vi "TCP SSH.vi"(6 "States":T1, 7 "Error In":errorcluster) -> (0 "Error  Out":errorcluster, 2 "Response":string)   [LabVIEW 2021]
uses:
  TCP states.ctl
  <vilib>/Field R&D Services/LIBSSH2 for LabVIEW/Toolkit/Session/Support/Create from SSH.vi
  <vilib>/Field R&D Services/LIBSSH2 for LabVIEW/Toolkit/Session/Support/Password Authentication.vi
  <vilib>/Field R&D Services/LIBSSH2 for LabVIEW/Toolkit/Channel/Support/Create from Session.vi
  <vilib>/Field R&D Services/LIBSSH2 for LabVIEW/Toolkit/Channel/Support/Destroy to Session.vi
  <vilib>/Field R&D Services/LIBSSH2 for LabVIEW/Toolkit/Session/Support/Destroy to SSH.vi
  <vilib>/Field R&D Services/LIBSSH2 for LabVIEW/Toolkit/Channel/Channel.lvclass
  <vilib>/Field R&D Services/LIBSSH2 for LabVIEW/Toolkit/SSH/SSH.lvclass
  <vilib>/Field R&D Services/LIBSSH2 for LabVIEW/Toolkit/Session/Session.lvclass
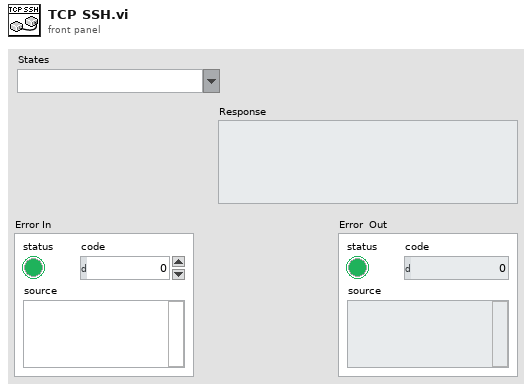
[diagram p1: front panel]
types:
  T1 = typedef "TCP states.ctl" = string
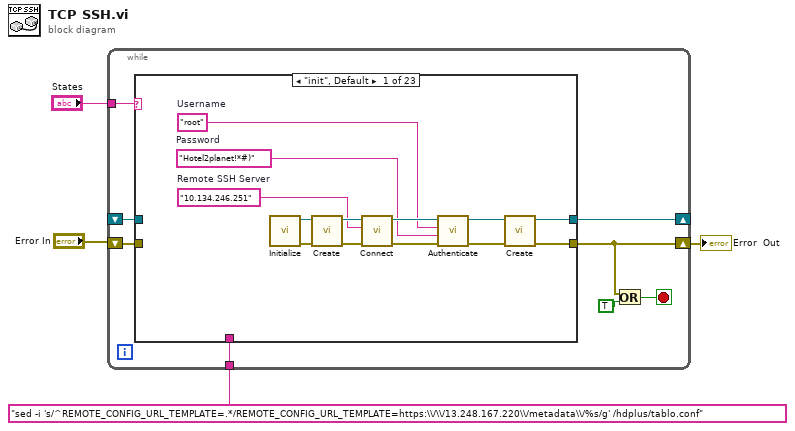
[diagram p0: block diagram]
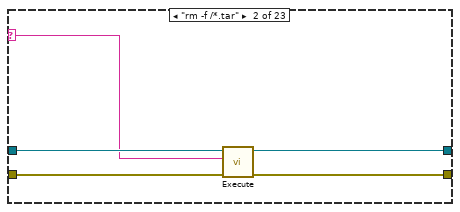
[diagram p2: hidden frame]
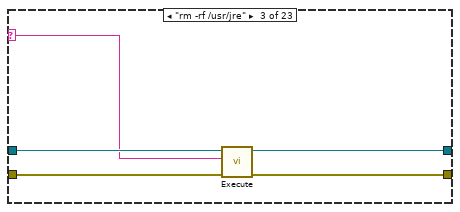
[diagram p3: hidden frame]
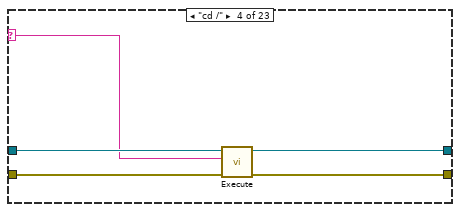
[diagram p4: hidden frame]
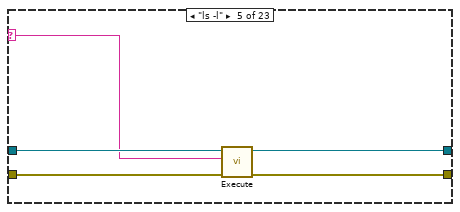
[diagram p5: hidden frame]
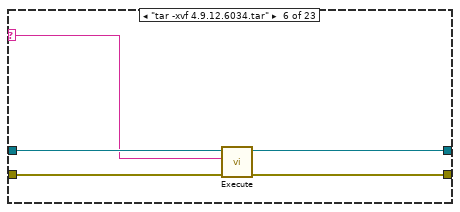
[diagram p6: hidden frame]
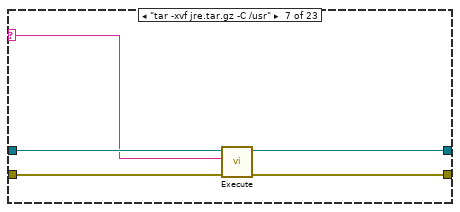
[diagram p7: hidden frame]
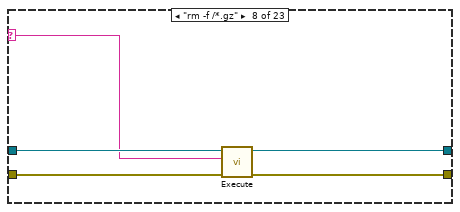
[diagram p8: hidden frame]
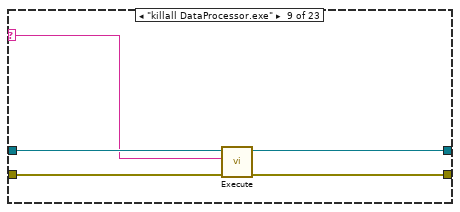
[diagram p9: hidden frame]
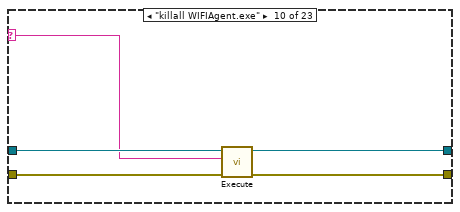
[diagram p10: hidden frame]
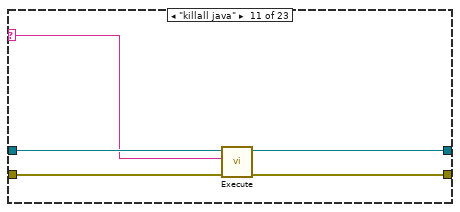
[diagram p11: hidden frame]
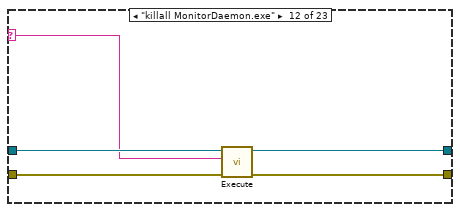
[diagram p12: hidden frame]
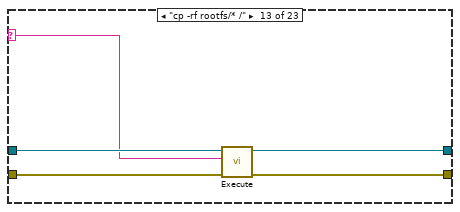
[diagram p13: hidden frame]
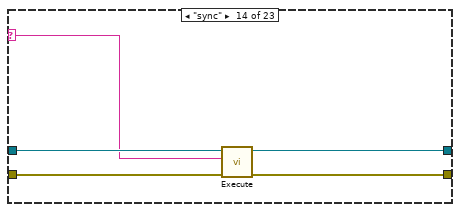
[diagram p14: hidden frame]
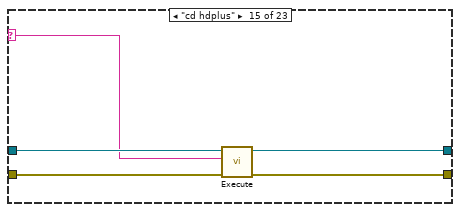
[diagram p15: hidden frame]
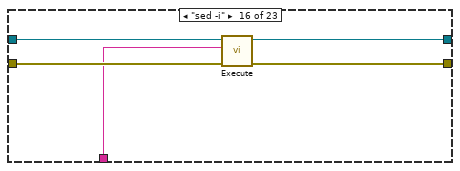
[diagram p16: hidden frame]
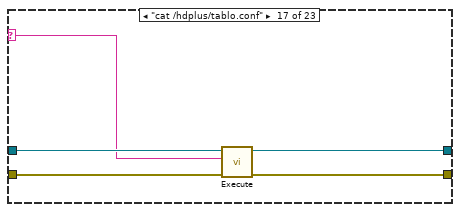
[diagram p17: hidden frame]
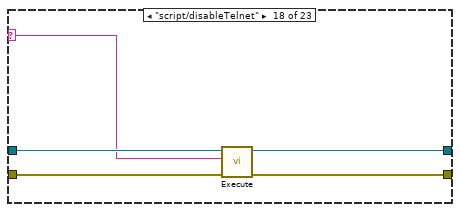
[diagram p18: hidden frame]
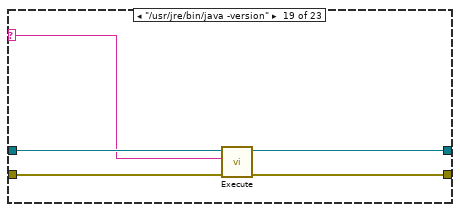
[diagram p19: hidden frame]
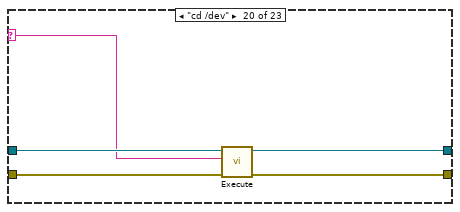
[diagram p20: hidden frame]
diagram:
  n1 = while {
    tunnel: "States" -> [w12]
    shift-right: [w10] -> _
    shift-left: _ -> [w11]
    shift-right: [w8] -> w2
    shift-left: "Error In" -> [w9]
    tunnel: "sed -i 's/^REMOTE_CONFIG_URL_TEMPLATE=.*/REMOTE_CONFIG_URL_TEMPLATE=https:\\/\\/13.248.167.220\\/metadata\\/%s/g' /hdplus/tablo.conf" ("Command") -> [w5]
    stop <- w6 stop-if-true
    n2 = case shown="\"init\", Default" w12 {
      selector: w12 -> [_ w28 w33 w38 w43 w48 w53 w58 w63 w68 w73 w78 w83 w88 w93 _ w101 w106 w111 w116 w121 _ _]
      tunnel: w11 -> [_ w30 w35 w40 w45 w50 w55 w60 w65 w70 w75 w80 w85 w90 w95 w100 w105 w110 w115 w120 w125 w128 w135]
      tunnel: [w15 w29 w32 w37 w42 w47 w52 w57 w62 w67 w72 w77 w82 w87 w92 w98 w103 w108 w113 w118 w123 w126 _] -> w10
      tunnel: [w13 w26 w31 w36 w41 w46 w51 w56 w61 w66 w71 w76 w81 w86 w91 w97 w102 w107 w112 w117 w122 w127 w133] -> w8
      tunnel: w9 -> [_ w27 w34 w39 w44 w49 w54 w59 w64 w69 w74 w79 w84 w89 w94 w99 w104 w109 w114 w119 w124 w129 w134]
      tunnel: w5 -> [_ _ _ _ _ _ _ _ _ _ _ _ _ _ _ w96 _ _ _ _ _ _ _]
      frame "init", Default {
        w17 = "10.134.246.251"  # Remote SSH Server
        w19 = "Hotel2planet!*#)"  # Password
        w18 = "root"  # Username
        n3 = call <vilib>:"Initialize.vi"() -> ("Error Out"=w21:errorcluster, "SSH"=w20:refnum<class "SSH.lvclass">)  [unwired: 10 in]
        n4 = call-poly <vilib>:"Create.vi"("Error In"=w21, "SSH"=w20) -> ("Error Out"=w23:errorcluster, "Sesssion"=w22:refnum<class "Session.lvclass">)  [unwired: 8 in]
        n5 = call <vilib>:"Connect.vi"("Error In"=w23, "Address"=w17, "Session In"=w22) -> ("Error Out"=w25:errorcluster, "Sesssion Out"=w24:refnum<class "Session.lvclass">)  [unwired: 7 in]
        n6 = call-poly <vilib>:"Authenticate.vi"("Error In"=w25, "Password"=w19, "Username"=w18, "Session In"=w24) -> ("Error Out"=w14:errorcluster, "Sesssion Out"=w16:refnum<class "Session.lvclass">)  [unwired: 6 in]
        n7 = call-poly <vilib>:"Create.vi"("Error In"=w14, "Session"=w16) -> ("Error Out"=w13:errorcluster, "Channel"=w15:refnum<class "Channel.lvclass">)  [unwired: 8 in]
      }
      frame "rm -f /*.tar" {
        n8 = call <vilib>:"Execute.vi"("Error In"=w27, "Command"=w28, "Channel In"=w30) -> ("Error Out"=w26:errorcluster, "Channel Out"=w29:refnum<class "Channel.lvclass">)  [unwired: 7 in]
      }
      frame "rm -rf /usr/jre" {
        n9 = call <vilib>:"Execute.vi"("Error In"=w34, "Command"=w33, "Channel In"=w35) -> ("Error Out"=w31:errorcluster, "Channel Out"=w32:refnum<class "Channel.lvclass">)  [unwired: 7 in]
      }
      frame "cd /" {
        n10 = call <vilib>:"Execute.vi"("Error In"=w39, "Command"=w38, "Channel In"=w40) -> ("Error Out"=w36:errorcluster, "Channel Out"=w37:refnum<class "Channel.lvclass">)  [unwired: 7 in]
      }
      frame "ls -l" {
        n11 = call <vilib>:"Execute.vi"("Error In"=w44, "Command"=w43, "Channel In"=w45) -> ("Error Out"=w41:errorcluster, "Channel Out"=w42:refnum<class "Channel.lvclass">)  [unwired: 7 in]
      }
      frame "tar -xvf 4.9.12.6034.tar" {
        n12 = call <vilib>:"Execute.vi"("Error In"=w49, "Command"=w48, "Channel In"=w50) -> ("Error Out"=w46:errorcluster, "Channel Out"=w47:refnum<class "Channel.lvclass">)  [unwired: 7 in]
      }
      frame "tar -xvf jre.tar.gz -C /usr" {
        n13 = call <vilib>:"Execute.vi"("Error In"=w54, "Command"=w53, "Channel In"=w55) -> ("Error Out"=w51:errorcluster, "Channel Out"=w52:refnum<class "Channel.lvclass">)  [unwired: 7 in]
      }
      frame "rm -f /*.gz" {
        n14 = call <vilib>:"Execute.vi"("Error In"=w59, "Command"=w58, "Channel In"=w60) -> ("Error Out"=w56:errorcluster, "Channel Out"=w57:refnum<class "Channel.lvclass">)  [unwired: 7 in]
      }
      frame "killall DataProcessor.exe" {
        n15 = call <vilib>:"Execute.vi"("Error In"=w64, "Command"=w63, "Channel In"=w65) -> ("Error Out"=w61:errorcluster, "Channel Out"=w62:refnum<class "Channel.lvclass">)  [unwired: 7 in]
      }
      frame "killall WIFIAgent.exe" {
        n16 = call <vilib>:"Execute.vi"("Error In"=w69, "Command"=w68, "Channel In"=w70) -> ("Error Out"=w66:errorcluster, "Channel Out"=w67:refnum<class "Channel.lvclass">)  [unwired: 7 in]
      }
      frame "killall java" {
        n17 = call <vilib>:"Execute.vi"("Error In"=w74, "Command"=w73, "Channel In"=w75) -> ("Error Out"=w71:errorcluster, "Channel Out"=w72:refnum<class "Channel.lvclass">)  [unwired: 7 in]
      }
      frame "killall MonitorDaemon.exe" {
        n18 = call <vilib>:"Execute.vi"("Error In"=w79, "Command"=w78, "Channel In"=w80) -> ("Error Out"=w76:errorcluster, "Channel Out"=w77:refnum<class "Channel.lvclass">)  [unwired: 7 in]
      }
      frame "cp -rf rootfs/* /" {
        n19 = call <vilib>:"Execute.vi"("Error In"=w84, "Command"=w83, "Channel In"=w85) -> ("Error Out"=w81:errorcluster, "Channel Out"=w82:refnum<class "Channel.lvclass">)  [unwired: 7 in]
      }
      frame "sync" {
        n20 = call <vilib>:"Execute.vi"("Error In"=w89, "Command"=w88, "Channel In"=w90) -> ("Error Out"=w86:errorcluster, "Channel Out"=w87:refnum<class "Channel.lvclass">)  [unwired: 7 in]
      }
      frame "cd hdplus" {
        n21 = call <vilib>:"Execute.vi"("Error In"=w94, "Command"=w93, "Channel In"=w95) -> ("Error Out"=w91:errorcluster, "Channel Out"=w92:refnum<class "Channel.lvclass">)  [unwired: 7 in]
      }
      frame "sed -i" {
        n22 = call <vilib>:"Execute.vi"("Error In"=w99, "Command"=w96, "Channel In"=w100) -> ("Error Out"=w97:errorcluster, "Channel Out"=w98:refnum<class "Channel.lvclass">)  [unwired: 7 in]
      }
      frame "cat /hdplus/tablo.conf" {
        n23 = call <vilib>:"Execute.vi"("Error In"=w104, "Command"=w101, "Channel In"=w105) -> ("Error Out"=w102:errorcluster, "Channel Out"=w103:refnum<class "Channel.lvclass">)  [unwired: 7 in]
      }
      frame "script/disableTelnet" {
        n24 = call <vilib>:"Execute.vi"("Error In"=w109, "Command"=w106, "Channel In"=w110) -> ("Error Out"=w107:errorcluster, "Channel Out"=w108:refnum<class "Channel.lvclass">)  [unwired: 7 in]
      }
      frame "/usr/jre/bin/java -version" {
        n25 = call <vilib>:"Execute.vi"("Error In"=w114, "Command"=w111, "Channel In"=w115) -> ("Error Out"=w112:errorcluster, "Channel Out"=w113:refnum<class "Channel.lvclass">)  [unwired: 7 in]
      }
      frame "cd /dev" {
        n26 = call <vilib>:"Execute.vi"("Error In"=w119, "Command"=w116, "Channel In"=w120) -> ("Error Out"=w117:errorcluster, "Channel Out"=w118:refnum<class "Channel.lvclass">)  [unwired: 7 in]
      }
      frame "ls sd* -l" {
        n27 = call <vilib>:"Execute.vi"("Error In"=w124, "Command"=w121, "Channel In"=w125) -> ("Error Out"=w122:errorcluster, "Channel Out"=w123:refnum<class "Channel.lvclass">)  [unwired: 7 in]
      }
      frame "Read" {
        n28 = call <vilib>:"Read.vi"("Error In"=w129, "Max Data Length"=u64 32000, "Channel In"=w128) -> ("Error Out"=w127:errorcluster, "Data"=w132:u8[], "Channel Out"=w126:refnum<class "Channel.lvclass">)  [unwired: 6 in]
        n29 = Byte Array To String(unsigned byte array=w132) -> (string=→"Response":string)
      }
      frame "Close" {
        n30 = call <vilib>:"Send Done.vi"("Error In"=w134, "Channel In"=w135) -> ("Error Out"=w137:errorcluster, "Channel Out"=w136:refnum<class "Channel.lvclass">)  [unwired: 8 in]
        n31 = call-poly <vilib>:"Destroy.vi"("Error In"=w137, "Channel"=w136) -> ("Error Out"=w139:errorcluster, "Session"=w138:refnum<class "Session.lvclass">)  [unwired: 8 in]
        n32 = call <vilib>:"Disconnect.vi"("Error In"=w139, "Session In"=w138) -> ("Error Out"=w141:errorcluster, "Sesssion Out"=w140:refnum<class "Session.lvclass">)  [unwired: 8 in]
        n33 = call-poly <vilib>:"Destroy.vi"("Error In"=w141, "Session"=w140) -> ("Error Out"=w143:errorcluster, "SSH"=w142:refnum<class "SSH.lvclass">)  [unwired: 8 in]
        n34 = call <vilib>:"Shutdown.vi"("Error In"=w143, "SSH"=w142) -> ("Error Out"=w133:errorcluster)  [unwired: 9 in]
      }
    }
    n35 = Or(x=w8, y=TRUE) -> (x .or. y?=w6:bool)
  }
  "Error  Out" <- w2
